vi "MCL DLL Version.vi"(10 "revision":i16, 11 "version":i16) -> (2 "revision out":i16, 3 "version out":i16)   [LabVIEW 2017, in "Madlib.lvlib"]
doc: "MADLIB_API void MCL_DLLVersion(short *version, short *revision);"
uses:
  Madlib.lvlib
  Madlib.dll
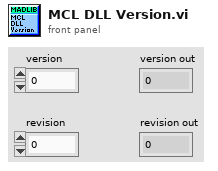
[diagram p1: front panel]
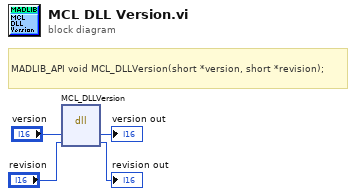
[diagram p0: block diagram]
diagram:
  # "MADLIB_API\tvoid\tMCL_DLLVersion(short *version, short *revision);"
  n1 = dll-call lib="C:/Users/francesco/dev/pump-probe/Piezo/lvlib/Madlib.*" fn="MCL_DLLVersion"("version"="version", "revision"="revision") -> ("version"=→"version out":i16, "revision"=→"revision out":i16)  [unwired: 4 in, 2 out]
